vi "Right Click.vi"(8 "error in (no error)":errorcluster, 11 "column in":refnum<class "Column.lvclass">) -> (0 "error out":errorcluster, 3 "column out":refnum<class "Column.lvclass">)   [LabVIEW 2014, in "Table Manager.lvlib" / "Column.lvclass"]
uses:
  Column.lvclass
  Table Manager/Menu Select.ctl
  Table Manager/Table Manager.lvclass
panel:
  in  "Menu Selection":refnum<user-event>
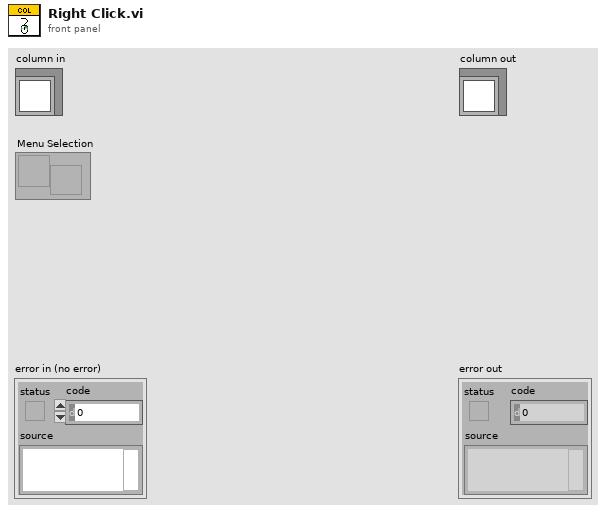
[diagram p1: front panel]
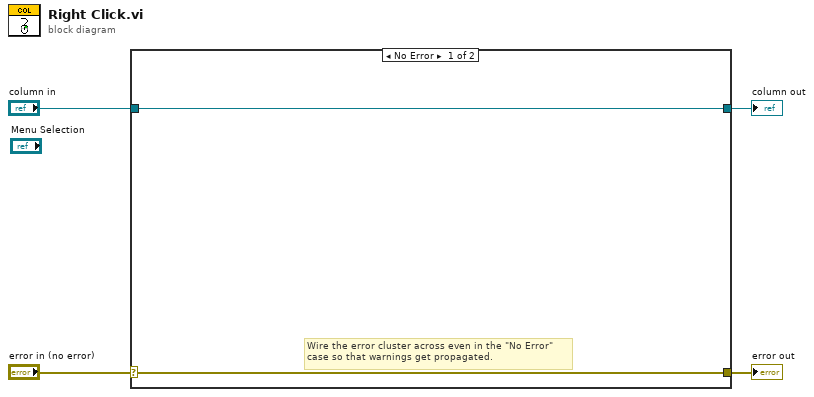
[diagram p0: block diagram]
diagram:
  n1 = case shown="No Error" "error in (no error)" {
    selector: "error in (no error)" -> [w5 w8]
    tunnel: [w5 w8] -> w3
    tunnel: [w6 w7] -> w1
    tunnel: "column in" -> [w6 w7]
    frame No Error {
      # "Wire the error cluster across even in the \"No Error\"\ncase so that warnings get propagated."
    }
    frame Error {
    }
  }
  "error out" <- w3
  "column out" <- w1
